vi "CreateVIA.vi"() -> (3 "VIA.lvclass":refnum<class "VIA.lvclass">)   [LabVIEW 2012, in "VIA.lvclass"]
uses:
  <vilib>/NXT/LegoClasses/VIA/VIA.lvclass
  <vilib>/NXT/NXT Controls/ConnectionType.ctl
  <vilib>/NXT/LegoClasses/MINDSTORMS/Write User Visible Name.vi
  <vilib>/NXT/LegoClasses/MINDSTORMS/Write Connection Type.vi
  <vilib>/NXT/LegoClasses/MINDSTORMS/Write Resource String.vi
  <vilib>/NXT/LegoClasses/MINDSTORMS/Write BT Address.vi
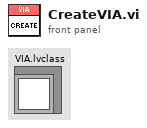
[diagram p1: front panel]
types:
  T1 = typedef "ConnectionType.ctl" = enum16{"Bluetooth", "USB", "WiFi"}
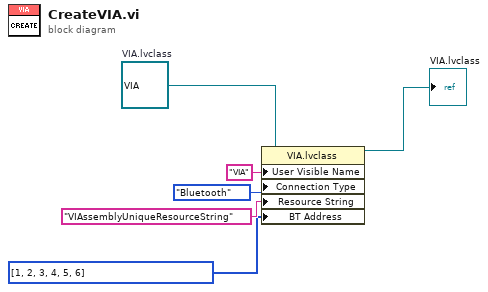
[diagram p0: block diagram]
diagram:
  w6 = refnum<class "VIA.lvclass"> refnum  # VIA.lvclass
  n1 = property class="VIA.lvclass"(reference=w6, "User Visible Name"="VIA", "Connection Type"=ConnectionType."Bluetooth", "Resource String"="VIAssemblyUniqueResourceString", "BT Address"=u8[] [1, 2, 3, 4, 5, 6]) -> (reference out=→"VIA.lvclass":refnum<class "VIA.lvclass">)  [unwired: 1 in, 1 out]
